vi "AuMT8852B Status Byte Query.vi"(8 "error in (no error)":errorcluster, 11 "VISA session":refnum<visa-resource-name>) -> (0 "error out":errorcluster, 2 "error code":i32, 3 "VISA session out":refnum<visa-resource-name>, 4 "Flags":T1 {"EUT Power State" items=["EUT power midrange", "EUT power max or min"]}, 6 "Status":i32)   [LabVIEW 2017]
doc: "Anritsu MT8852B Bluetooth Tester\n\nReturns the 8-bit Instrument Status Register, and clears the value in the instrument.\n\nBit 7 (most significant bit) -unused\n\nBit 6 - Request service - This bit is set (and an SRQ is generated) when one of the other bits in the status byte is set and the corresponding bit in the status register events (SRE) has been set.\n\nBit 5 - Message available - this bit is always set when there is data available to be read out of the output buffer and cleared when the output buffer is empty.\n\nBit 4 - Event status bit - this bit is set when a bit is set in the event register and the corresponding bit has been set in the event status enable register (ESE).\n\nBit 3 - Event status bit - this bit is set when a bit is set in the event register and the corresponding bit has been set in the event status enable register (ESE).\n\nBit 2 - EUT Power State - This bit is set when the EUT is at either max or min power.\n\nBit 1 - Equipment test fail - this bit is set when one of the equipment under test fail register bits has been set and the corresponding bit in the equipment under test fail register enable (ETE) bit has been set.\n\nBit 0 (least significant bit) - Instrument status - this bit is set when one of the instrument status bits has been set and the corresponding bit in the instrument status enable (INE) register has been set.\n\nOUTPUTS\nFlags - value of each status message contained in the register.\nStatus - integer value (0-255) of the register; in general, 0 means no error or event to report."
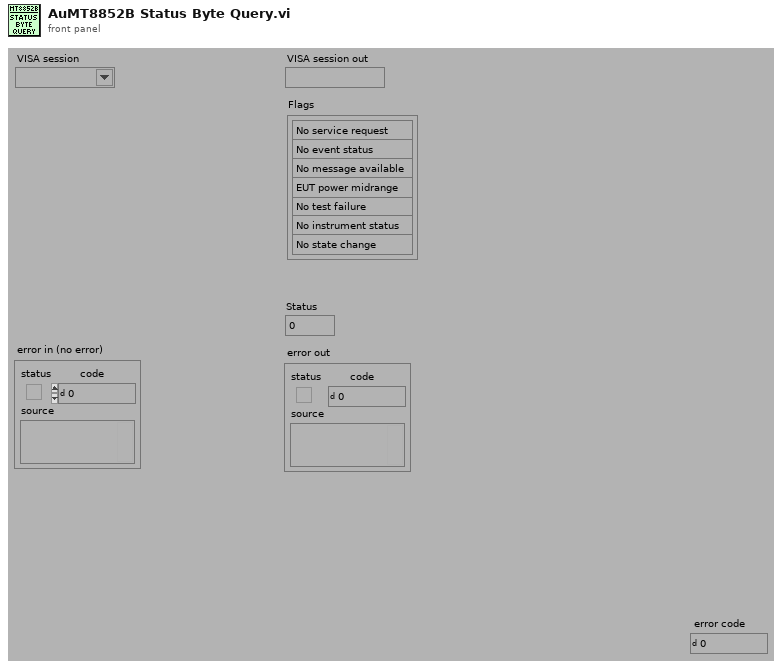
[diagram p1: front panel]
types:
  T1 = cluster{"Service request":enum16{"No service request", "Service request"}, "Event status":enum16{"No event status", "Event status"}, "Message":enum16{"No message available", "Message available"}, "Test failure":enum16{"No test failure", "Test failure"}, "Instrument status":enum16{"No instrument status", "Instrument status"}, "EUT Power State":u16, "State change":enum16{"No state change", "State change"}}
  T2 = enum16{"Simulate", "Range check", "Cache", "Query instrument status"}
  T3 = cluster{"[0]":i16, "[1]":i16, "[2]":i16, "[3]":i16, "[4]":i16, "[5]":i16, "[6]":i16, "[7]":i16}
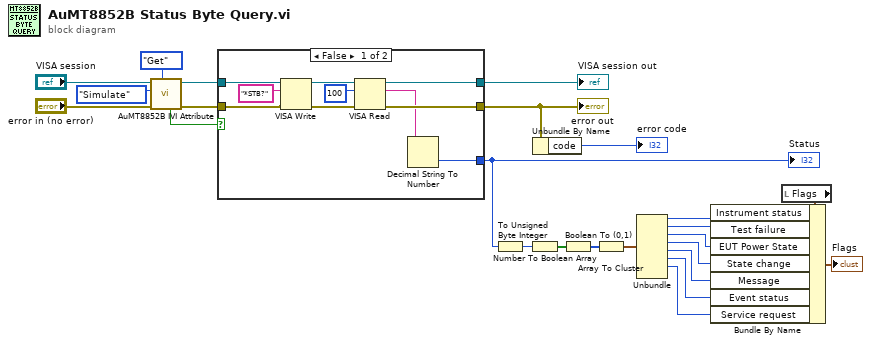
[diagram p0: block diagram]
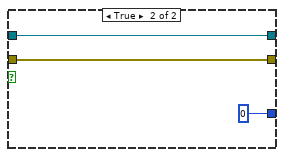
[diagram p2: hidden frame]
diagram:
  n1 = call <instrlib>:"AuMT8852B IVI Attribute.vi"("Set/Get (Set)"=enum16{"Set", "Get"}."Get", "error in (no error)"="error in (no error)", "Flag (Simulate)"=T2."Simulate", "VISA session"="VISA session") -> ("error out"=w21:errorcluster, "VISA session out"=w23:refnum<visa-resource-name>, "Value out"=w17:bool)  [unwired: 5 in]
  n2 = case shown="False" w17 {
    tunnel: [w30 w37] -> w24
    tunnel: [w29 w36] -> w8
    tunnel: [w25 u8 0] -> w15
    tunnel: w23 -> [w27 w37]
    tunnel: w21 -> [w26 w36]
    frame False {
      n3 = VISA Write(VISA resource name=w27, write buffer="*STB?" ("write buffer (\"\")"), error in (no error)=w26) -> (VISA resource name out=w33:refnum<visa-resource-name>, error out=w32:errorcluster)  [unwired: 1 out]
      n4 = VISA Read(VISA resource name=w33, byte count=u32 100 ("byte count (0)"), error in (no error)=w32) -> (VISA resource name out=w30:refnum<visa-resource-name>, read buffer=w28:string, error out=w29:errorcluster)  [unwired: 1 out]
      n5 = Decimal String To Number(string=w28) -> (number=w25:i32)  [unwired: 2 in, 1 out]
    }
    frame True {
    }
  }
  "error out" <- w8
  "VISA session out" <- w24
  "Status" <- w15
  n6 = To Unsigned Byte Integer(number=w15) -> (unsigned 8bit integer=w14:u8)
  n7 = Number To Boolean Array(number=w14) -> (Boolean array=w13:bool[])
  n8 = Unbundle By Name(w8) -> ("code"=→"error code":i32)
  n9 = Boolean To (0,1)(Boolean=w13) -> (0, 1=w12:i16[])
  n10 = Array To Cluster(array=w12) -> (cluster=w11:T3)
  n11 = Unbundle(w11) -> ("[0]"=w7:i16, "[1]"=w6:i16, "[2]"=w5:i16, "[3]"=w1:i16, "[4]"=w4:i16, "[5]"=w3:i16, "[6]"=w2:i16)  [unwired: 1 out]
  n12 = local read "Flags"() -> (w16:T1)
  n13 = Bundle By Name(cluster=w16, "Instrument status"=w7, "Test failure"=w6, "EUT Power State"=w5, "State change"=w1, "Message"=w4, "Event status"=w3, "Service request"=w2) -> (→"Flags":T1)
